vi "Front Arm Positions.vi"() -> (2 "Rear Arm":T1={"Down"=0.82, "Pickup"=0.72, "Shoot"=0.7, "Turtle"=0.38, "Intake Block"=0.4, "Intake Transfer"=0.42, "Cheval De Fris"=0.52, "Hang"=0.58}, 3 "Front Arm":T2={"Down"=0.71, "Pickup"=0.675, "Shoot"=0.58, "Turtle"=0.29, "Intake Transfer"=0.37, "Hang"=0.595})   [LabVIEW 2015, in "ArmController.lvlib"]
uses:
  ArmController/ArmController.lvlib
panel:
  in  "Practice Bot Rear Arm":T1={"Down"=0.82, "Pickup"=0.715, "Shoot"=0.7, "Turtle"=0.38, "Intake Block"=0.5, "Intake Transfer"=0.42, "Cheval De Fris"=0.608, "Hang"=0.52}
  in  "Practice Bot Front Arm":T2={"Down"=0.71, "Pickup"=0.658, "Shoot"=0.52, "Turtle"=0.29, "Intake Transfer"=0.37, "Hang"=0.52}
  in  "Rear Arm":T1={"Down"=0.82, "Pickup"=0.72, "Shoot"=0.7, "Turtle"=0.38, "Intake Block"=0.4, "Intake Transfer"=0.42, "Cheval De Fris"=0.52, "Hang"=0.58}
  in  "Front Arm":T2={"Down"=0.71, "Pickup"=0.675, "Shoot"=0.58, "Turtle"=0.29, "Intake Transfer"=0.37, "Hang"=0.595}
  # ".675 -->"
  # "Final Bot"
  # "Practice Bot"
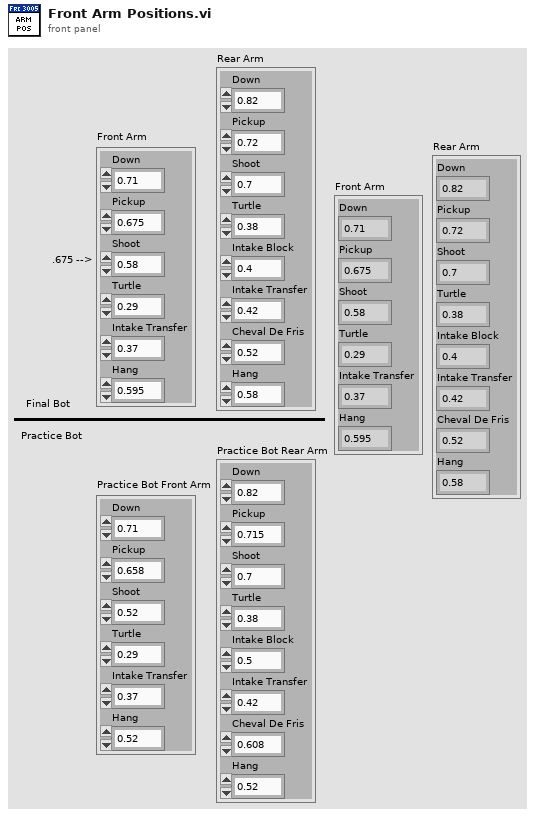
[diagram p1: front panel]
types:
  T1 = cluster{"Down":dbl, "Pickup":dbl, "Shoot":dbl, "Turtle":dbl, "Intake Block":dbl, "Intake Transfer":dbl, "Cheval De Fris":dbl, "Hang":dbl}
  T2 = cluster{"Down":dbl, "Pickup":dbl, "Shoot":dbl, "Turtle":dbl, "Intake Transfer":dbl, "Hang":dbl}
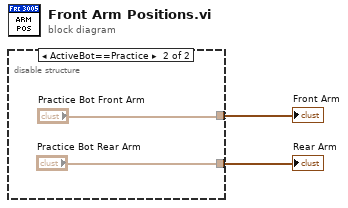
[diagram p0: block diagram]
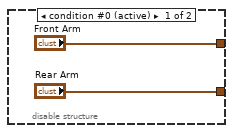
[diagram p2: hidden frame]
diagram:
  n1 = disable-structure shown="ActiveBot==Practice" {
    disable-tunnel: ["Front Arm" "Practice Bot Front Arm"] -> w2
    disable-tunnel: ["Rear Arm" "Practice Bot Rear Arm"] -> w1
    frame condition #0 (active) {
    }
    frame condition #1 {
    }
  }
  "Front Arm" <- w2
  "Rear Arm" <- w1
